vi "数据队列（U8）.vi"(7 "init":bool caption="初始化", 10 "length":i32=100 caption="采样长度", 11 "input":u8 caption="输入数据点") -> (1 "Previous Queue":u8[](array[numeric]) caption="之前队列", 2 "Current Queue":u8[](array[numeric]) caption="当前队列", 3 "eliminated":u8 caption="已除去的元素", 4 "current length":i32 caption="当前长度")   [LabVIEW 2011]
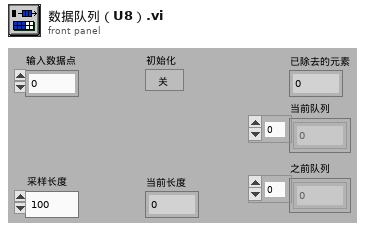
[diagram p1: front panel]
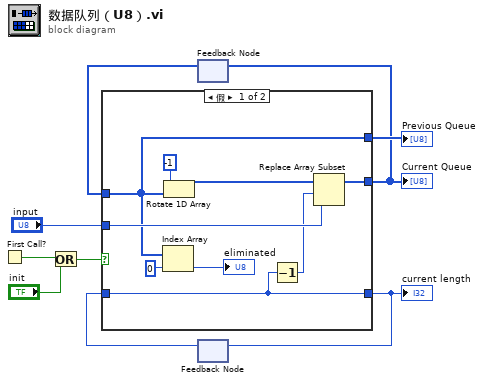
[diagram p0: block diagram]
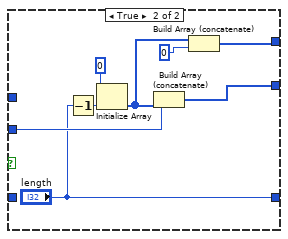
[diagram p2: hidden frame]
diagram:
  n1 = First Call?() -> (First Call?: T/F=w3:bool)
  n2 = Or(x=w3, y="init") -> (x .or. y?=w4:bool)
  n3 = feedback #1() -> (w7:u8[])  [unwired: 1 in]
  n4 = feedback #2() -> (w8:i32)  [unwired: 1 in]
  n5 = case shown="假" w4 {
    tunnel: [w16 w20] -> w2
    tunnel: [w11 "length"] -> w1
    tunnel: w8 -> [w11 _]
    tunnel: w7 -> [w13 _]
    tunnel: "input" -> [w17 w26]
    tunnel: [w13 w21] -> w9
    frame False {
      n6 = Index Array(array=w13, index=0 ("Index")) -> (element=→"eliminated":u8)
      n7 = Rotate 1D Array(1:w13, 2:i16 -1 ("n")) -> (0:w14:u8[])
      n8 = Decrement(x=w11) -> (x-1=w10:i32)
      n9 = Replace Array Subset(array=w14, new element=w17, index=w10) -> (w16:u8[])
    }
    frame True {
      n10 = Decrement(x="length") -> (x-1=w25:i32)
      n11 = Initialize Array(u8 0 ("Element Data"), w25) -> (w23:u8[])
      n12 = Build Array (concatenate)(w23, w26) -> (w20:u8[])
      n13 = Build Array (concatenate)(w23, u8 0 ("Input Element")) -> (w21:u8[])
    }
  }
  "Current Queue" <- w2
  "current length" <- w1
  "Previous Queue" <- w9
  n14 = feedback-in #1(w2) -> ()
  n15 = feedback-in #2(w1) -> ()
